vi "TSM SSC DAQmx Reserve.vi"(0 "TSM DAQmx In":T1, 11 "error in (no error)":errorcluster) -> (4 "TSM DAQmx Out":T1, 15 "error out":errorcluster)   [LabVIEW 2020]
doc: "Calling this VI reserves the hardware resources needed for the task. No other tasks can reserve these same resources."
uses:
  Pin Map/TSM DAQmx Multi-Task.ctl
  <vilib>/NI_TestStand_SemiconductorModule/NI_TestStand_Semiconductor_Module.lvlibp/PinMap/PinQueryContext/MultiplePinMultipleSessionQueryContext/MultiplePinMultipleSessionQueryContext.lvclass
  Pin Map/SSC DAQmx.ctl
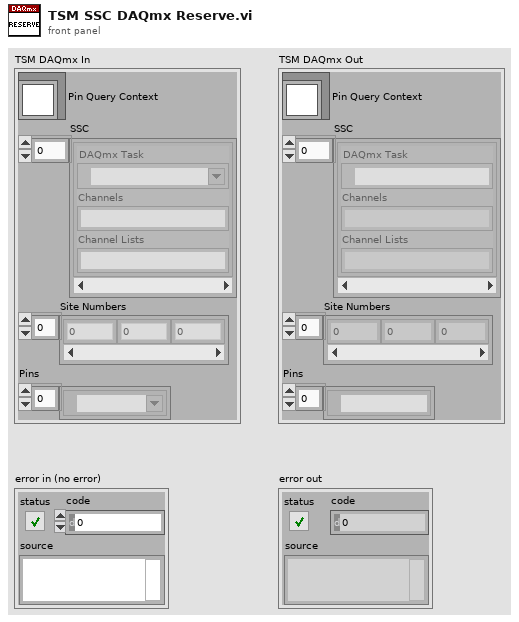
[diagram p1: front panel]
types:
  T1 = typedef "TSM DAQmx Multi-Task.ctl" = cluster{"Pin Query Context":refnum<class "MultiplePinMultipleSessionQueryContext.lvclass">, "SSC":T2[], "Site Numbers":i32[], "Pins":tag[]}
  T2 = typedef "SSC DAQmx.ctl" = cluster{"DAQmx Task ":refnum<k21>, "Channels":string, "Channel Lists":string}
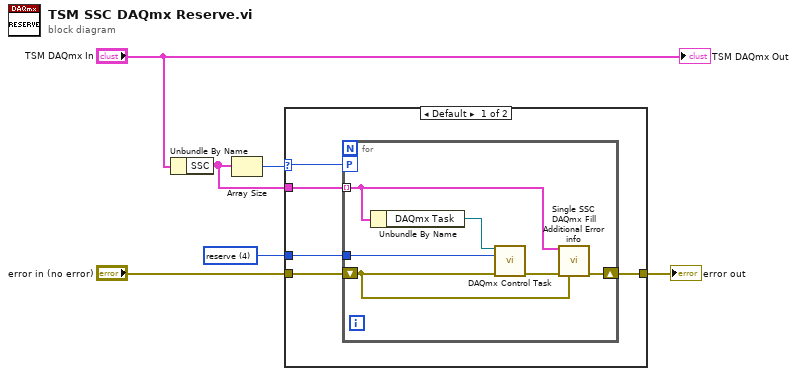
[diagram p0: block diagram]
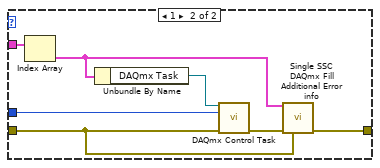
[diagram p2: hidden frame]
diagram:
  w1 = 4 items=["verify"=2, "reserve"=4, "commit"=3, "unreserve"=5, "abort"=6] ("action")
  n1 = Unbundle By Name("TSM DAQmx In") -> ("SSC"=w3:T2[])
  n2 = Array Size(array=w3) -> (size(s)=w2:i32)
  n3 = case shown="Default" w2 {
    selector: w2 -> [w9 _]
    tunnel: [w11 w23] -> w4
    tunnel: "error in (no error)" -> [w10 w21]
    tunnel: w3 -> [w8 w24]
    tunnel: w1 -> [w7 w18]
    frame Default {
      n4 = for {
        tunnel: w8 -> [w14] mode=indexing
        workers-P: w9 -> [_]
        shift-right: [w17] -> w11
        shift-left: w10 -> [w16]
        tunnel: w7 -> [w12]
        n5 = Unbundle By Name(w14) -> ("DAQmx Task"=w13:refnum<k21>)
        n6 = call <vilib>:"DAQmx Control Task.vi"("task/channels in"=w13, "action"=w12, "error in"=w16) -> ("error out"=w15:errorcluster)  [unwired: 11 in, 1 out]
        n7 = call "Single SSC DAQmx Fill Additional Error info.vi"("DAQmx SSC in"=w14, "error in"=w15, "previous error in"=w16) -> ("error out"=w17:errorcluster)  [unwired: 12 in]
      }
    }
    frame 1 {
      n8 = Index Array(array=w24) -> (element=w19:T2)  [unwired: 1 in]
      n9 = Unbundle By Name(w19) -> ("DAQmx Task"=w22:refnum<k21>)
      n10 = call <vilib>:"DAQmx Control Task.vi"("task/channels in"=w22, "action"=w18, "error in"=w21) -> ("error out"=w20:errorcluster)  [unwired: 11 in, 1 out]
      n11 = call "Single SSC DAQmx Fill Additional Error info.vi"("DAQmx SSC in"=w19, "error in"=w20, "previous error in"=w21) -> ("error out"=w23:errorcluster)  [unwired: 12 in]
    }
  }
  "error out" <- w4
  "TSM DAQmx Out" <- "TSM DAQmx In"
